vi "ROSNode.vi"(2 "Response":T1, 3 "ROS":T3={"topic port"=7000, "Node"="/LVROS", "topic"="/LVROS", "type"="", "node port"=7000, "error "={"status"=FALSE, "code"=0, "source"=""}, "Direction"=enum."Node", "Update (ms)"=1, "FIFO size"=1}) -> ()   [LabVIEW 2012]
doc: "Performs the functions of a ROS node: adds a publisher to the registered publisher list and registers with the master, starts and updates publishers, adds subscribers, and opens ports for subscribers and publishers"
uses:
  Console/Servers/ServerSubs/MyState.ctl
  _ROSDefinition.vi
  Console/Servers/ServerSubs/ROSLog.ctl
  <vilib>/Platform/browser.llb/Open URL in Default Browser (string).vi
  <vilib>/Utility/miscctls.llb/LVPointTypeDef.ctl
  SubVIs/_ROSDirection.ctl
  SubVIs/_ROSControl.ctl
panel:
  out "Color Code":picture
  out "Status out":T2[](array[typedef])
  out "Status":string
  out "Connections":bool
  out "Boundaries":cluster{i32, i32}[](array[cluster])=[{10, 22}, {30, 42}, {50, 62}]
  out "selection":i32=-1
  in  "HTML":bool
  out "ROS Master":string="130.64.16.138:11311"
  out "Registered":T3[](array[typedef])
  out "Last requestTopic":string
  out "Subscribers":T5(array[cluster])
  out "Queue log":string
  out "MyState":T2
  out "Setup":string
  in  "stop":bool
  out "HTML":picture
  out "Servers":picture
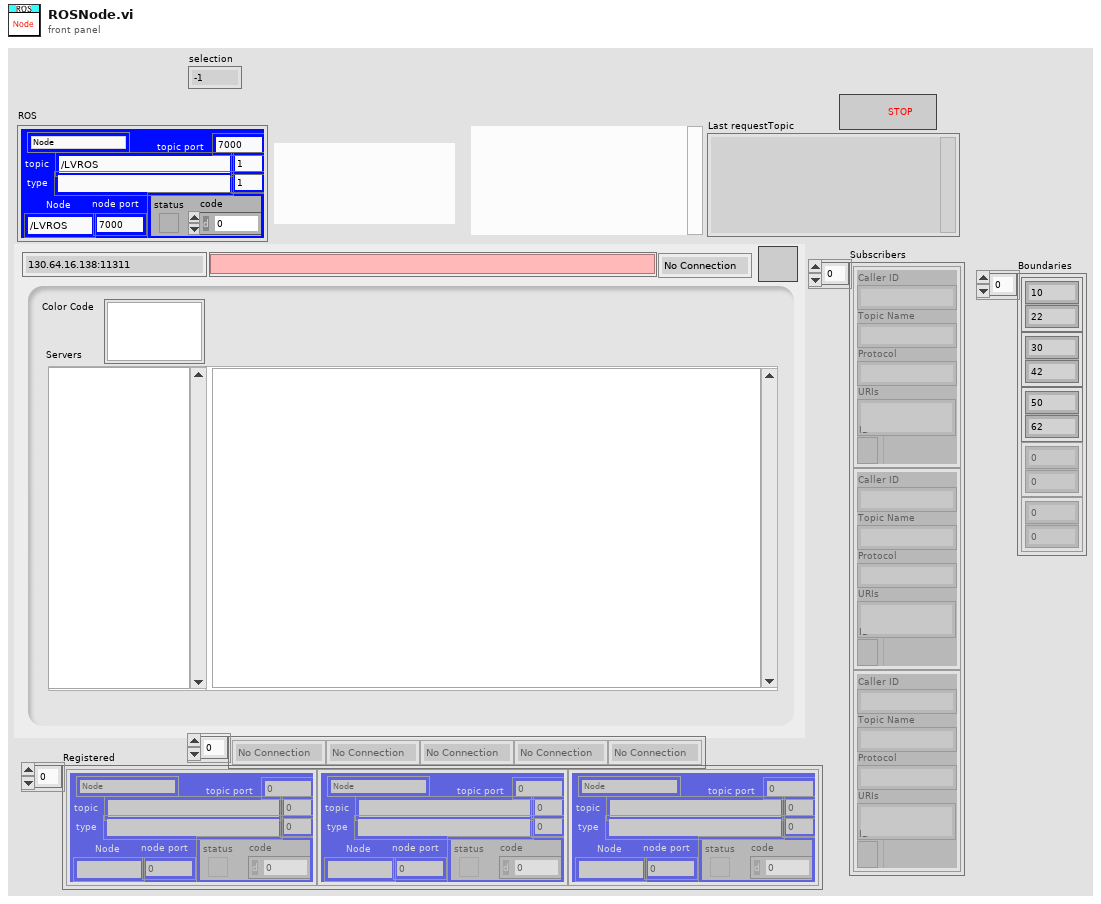
[diagram p1: front panel]
types:
  T1 = cluster{"Code":i32, "Status Message":string, "Nodes with this topic":string[]}
  T2 = typedef "MyState.ctl" = enum16{"No Connection", "Registered", "Connected", "Close"}
  T3 = typedef "_ROSControl.ctl" = cluster{"topic port":u16, "Node":string, "topic":string, "type":string, "node port":u16, "error ":errorcluster, "Direction":T4, "Update (ms)":u16, "FIFO size":u16}
  T4 = typedef "_ROSDirection.ctl" = enum16{"Node", "Publisher", "Subscriber", "ServiceClient", "ServiceProvider"}
  T5 = cluster{"Caller ID":string, "Topic Name":string, "Protocol":string, "URIs":string, "ID":refnum<k5>}[]
  T6 = enum16{"Reset Log", "Add Client", "Remove Client", "Add Task"}
  T7 = typedef "LVPointTypeDef.ctl" = cluster{"Horizontal":i16, "Vertical":i16}
  T8 = typedef "LVMouseTypeDef.ctl" = cluster{"Mouse Position":cluster{"X":i32, "Y":i32}, "Mouse Modifiers":cluster{"Button Down":bool, "Shift Mod":bool, "Menu Mod":bool, "Option Mod":bool}}
  T9 = cluster{"Caller ID":string, "Topic Name":string, "Node URIs":string[]}
  T10 = enum32{"Invalid", "Standard", "Closed", "Hidden", "Minimized", "Maximized"}
  T11 = typedef "ROSLog.ctl" = cluster{"Sent":string, "Reply":string, "MethodName":string, "success":bool, "Dir1":string, "Dir2":string, "Time Stamp":string, "error":errorcluster, "Preamble":string, "Midamble":string, "Postamble":string}
  T12 = cluster{"Caller ID":string, "Topic Name":string, "Protocol":string, "URI":string, "ID":refnum<k5>}
  T13 = cluster{"Caller ID":string, "Topic Name":string, "Protocol":string, "URI":string, "ID":refnum<k5>}[]
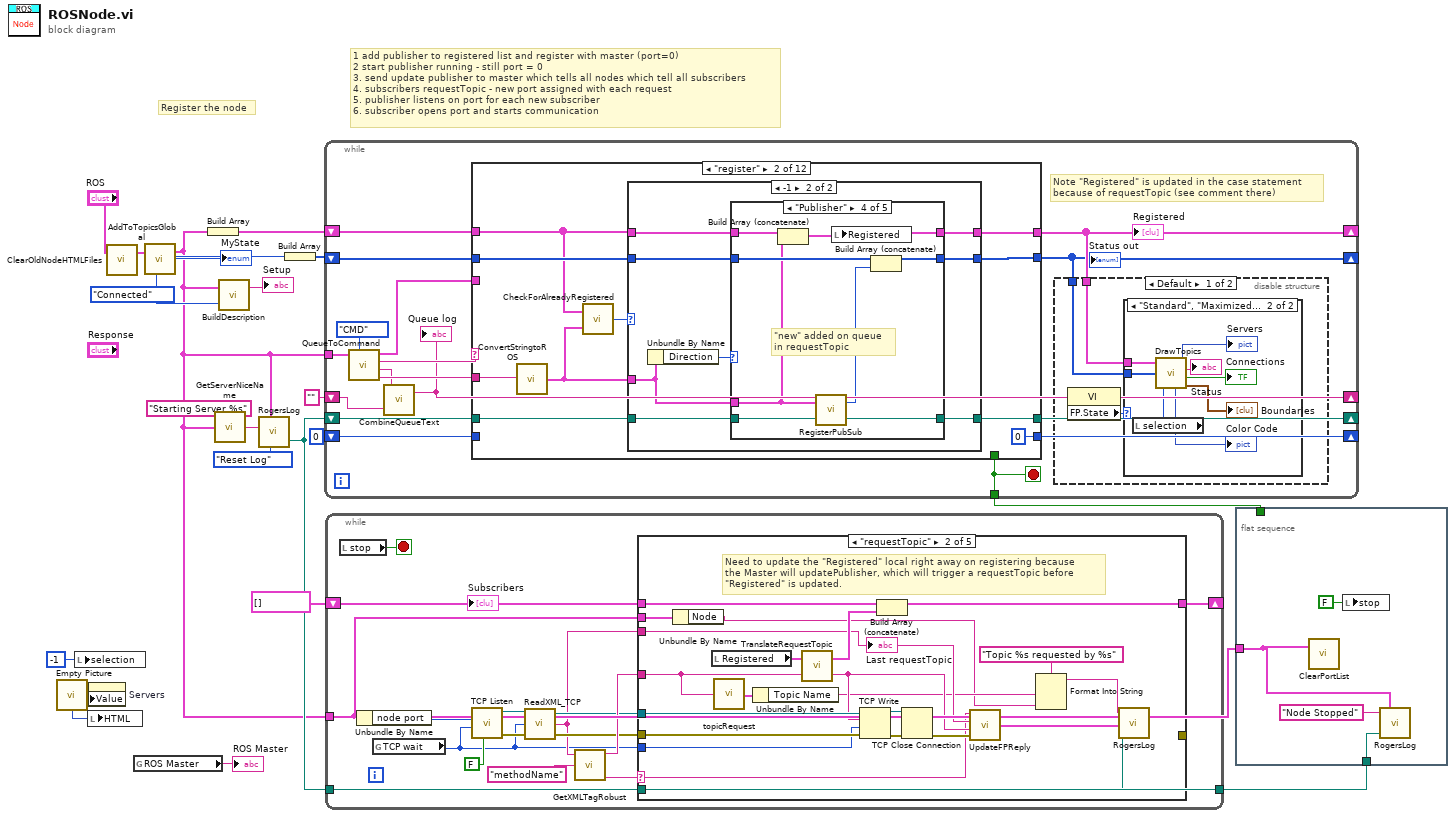
[diagram p0: block diagram]
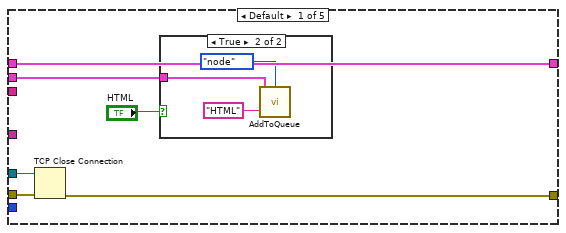
[diagram p2: hidden frame]
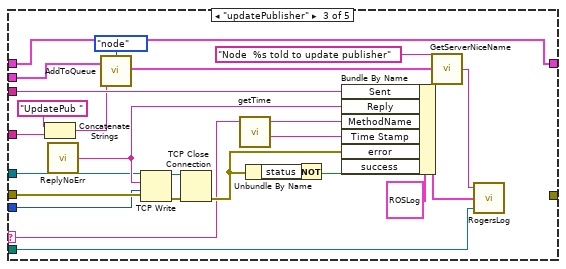
[diagram p4: hidden frame]
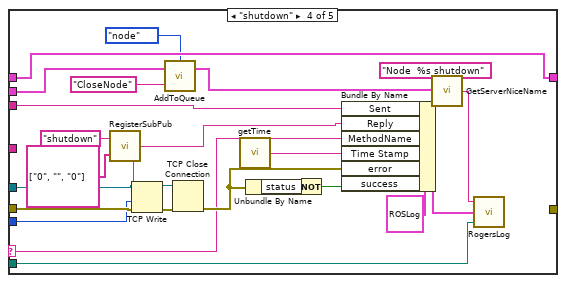
[diagram p5: hidden frame]
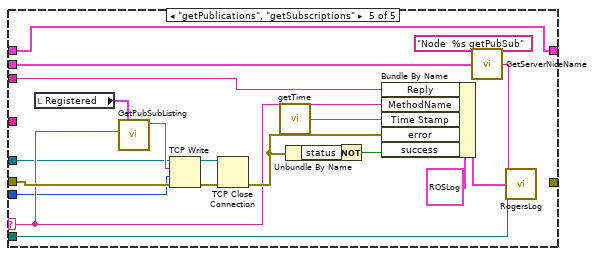
[diagram p6: hidden frame]
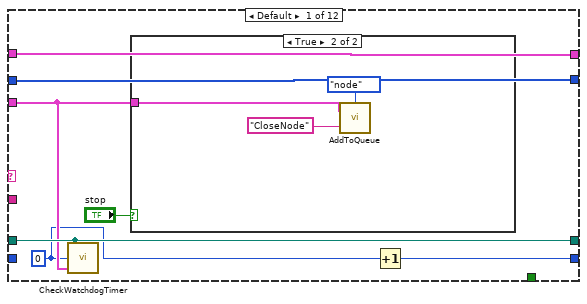
[diagram p9: hidden frame]
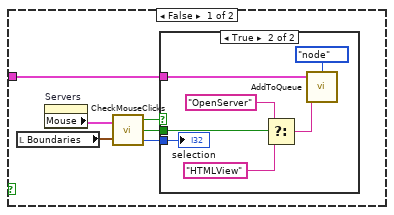
[diagram p10: hidden frame]
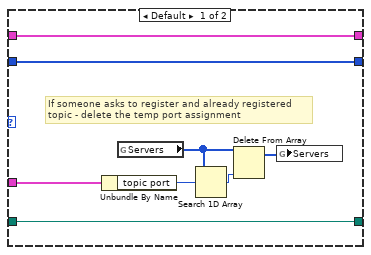
[diagram p12: hidden frame]
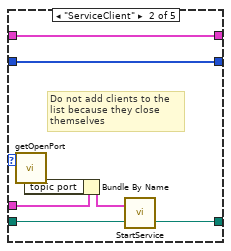
[diagram p14: hidden frame]
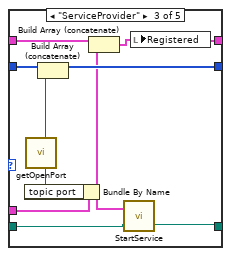
[diagram p15: hidden frame]
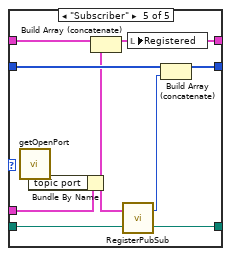
[diagram p16: hidden frame]
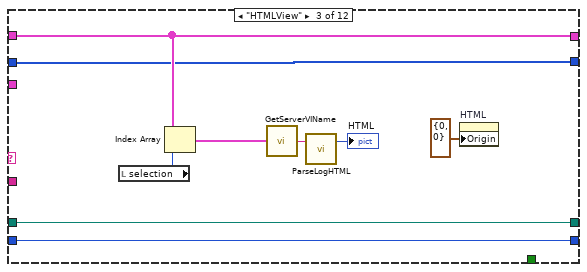
[diagram p17: hidden frame]
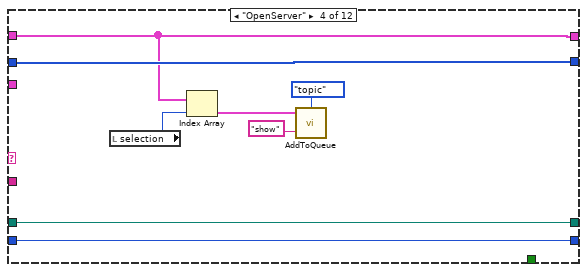
[diagram p18: hidden frame]
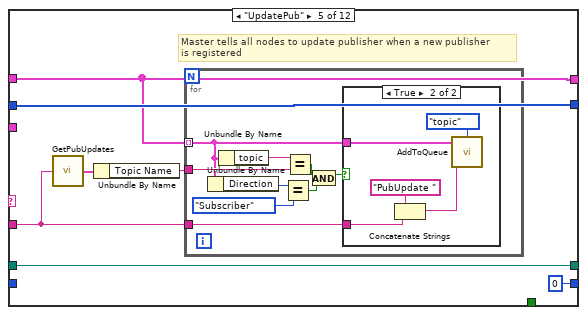
[diagram p19: hidden frame]
diagram:
  w12 = MyState."Connected" ("MyState")
  # "Register the node"
  # "1 add publisher to registered list and register with master (port=0)\n2 start publisher running - still port = 0\n3. send update publisher to master which tells all nodes which tell all subscribers\n4. subscribers requestTopic - new port assigned with each request\n5. publisher listens on port for each new subscriber\n6. subscriber opens port and starts communication"
  n1 = call "Empty Picture"() -> ("empty picture"=w10:picture)
  n2 = local write "selection"(-1 ("selection")) -> ()
  n3 = local write "HTML"(w10) -> ()
  n4 = property on="Servers" class="Pict"("Value"=w10) -> ()  [unwired: 2 in, 2 out]
  n5 = call "ClearOldNodeHTMLFiles.vi"("ROS"="ROS") -> ("ROS out"=w2:T3)  [unwired: 2 in]
  n6 = global read "_ROSDefinition.vi" "ROS Master"() -> (→"ROS Master":string)
  n7 = call "AddToTopicsGlobal.vi"("ROS in"=w2) -> ("ROS out"=w1:T3)  [unwired: 2 in]
  n8 = Build Array(w1) -> (w13:T3[])
  n9 = call "GetServerNiceName.vi"("ROS"=w1, "Text to add"="Starting Server %s") -> ("String"=w17:string)
  n10 = call "BuildDescription.vi"("MyState"=w12, "ROS in"=w1) -> ("Setup"=→"Setup":string)  [unwired: 1 in]
  n11 = call "RogersLog.vi"("Text to add"=w17, "ROS"=w1, "Task"=T6."Reset Log") -> ("LogPath out"=w7:path)  [unwired: 2 in, 1 out]
  n12 = Build Array(w12) -> (w11:T2[])
  n13 = while {
    tunnel: w1 -> [w30]
    tunnel: [w33] -> w14
    shift-right: [w29] -> _
    shift-left: w13 -> [w34]
    shift-right: [w31] -> _
    shift-left: w7 -> [w32]
    shift-right: [w27] -> _
    shift-left: w11 -> [w28]
    shift-right: [w25] -> _
    shift-left: 0 ("selection") -> [w26]
    shift-right: [w24] -> _
    shift-left: "" ("New List") -> [w23]
    stop <- w33 stop-if-true
    # "Note \"Registered\" is updated in the case statement\nbecause of requestTopic (see comment there)"
    n14 = call "QueueToCommand.vi"("ROS"=w30, "Check"=enum16{"Cmd+Write", "FIFO", "CMD", "CMD /wait"}."CMD") -> ("ROS out"=w21:T3, "Command"=w36:string, "Queue log"=w22:string, "data"=w35:string)  [unwired: 1 in]
    n15 = call "CombineQueueText.vi"("Old List"=w23, "Queue In"=w22) -> ("New List"=w24:string)  [unwired: 1 in]
    "Queue log" <- w24
    n16 = case shown="\"register\"" w36 {
      tunnel: w35 -> [_ w80 _ _ w152 w181 _ _ _ _ w239 _]
      tunnel: [w53 w79 w137 w148 w153 w175 w201 w209 w229 w233 w242 w261] -> w29
      tunnel: w34 -> [w53 w73 w137 w148 w153 w176 w202 w209 w229 w233 w242 w261]
      tunnel: [_ _ _ _ _ _ _ _ w226 _ _ _] -> w33
      tunnel: w32 -> [w51 w78 w139 w150 w157 w180 w204 w211 w227 w232 w248 w259]
      tunnel: [w51 w77 w139 w150 w157 w179 w204 w211 w227 w232 w248 w259] -> w31
      tunnel: w21 -> [w50 _ _ _ _ _ w196 w208 _ _ _ w257]
      tunnel: w28 -> [w52 w76 w135 w149 w156 w174 w200 w212 w228 w231 w245 w260]
      tunnel: [w52 w75 w135 w149 w156 w173 w199 w212 w228 w231 w244 w260] -> w27
      tunnel: w26 -> [_ _ w134 w146 _ _ _ _ w225 w230 _ w258]
      tunnel: [w49 0 w134 w146 0 0 0 0 w225 w230 0 ("selection") w258] -> w25
      frame Default {
        w48 = 0 ("selection")
        n17 = call "CheckWatchdogTimer.vi"("ROS"=w50, "itteration"=w48, "LogPath in"=w51) -> ()  [unwired: 3 in]
        n18 = case shown="True" "stop" {
          tunnel: w50 -> [w57 w69]
          frame False {
            n19 = local read "Boundaries"() -> (w56:cluster{i32, i32}[])
            n20 = property on="Servers" class="Pict"() -> ("Mouse"=w58:T8)  [unwired: 2 in, 2 out]
            n21 = call "CheckMouseClicks.vi"("Mouse"=w58, "Boundaries"=w56) -> ("Change?"=w59:bool, "Shift?"=w55:bool, "selection"=w60:i32)
            n22 = case shown="True" w59 {
              tunnel: w60 -> [_ w67]
              tunnel: w57 -> [_ w62]
              tunnel: w55 -> [_ w65]
              frame False {
              }
              frame True {
                n23 = Select(t="OpenServer" ("element"), s=w65, f="HTMLView" ("element")) -> (s? t:f=w63:string)
                n24 = call "AddToQueue.vi"("Cmd"=w63, "ROS"=w62, "Type"=enum16{"topic", "node", "ToFIFO", "ToWrite"}."node") -> ()  [unwired: 2 in, 1 out]
                "selection" <- w67
              }
            }
          }
          frame True {
            n25 = call "AddToQueue.vi"("Cmd"="CloseNode" ("element"), "ROS"=w69, "Type"=enum16{"topic", "node"}."node" ("Name")) -> ()  [unwired: 2 in, 1 out]
          }
        }
        n26 = Increment(x=w48) -> (x+1=w49:i32)
      }
      frame "register" {
        n27 = call "ConvertStringtoROS.vi"("string in"=w80) -> ("ROS"=w72:T3)
        n28 = call "CheckForAlreadyRegistered.vi"("ROS"=w72, "Registered"=w73) -> ("index of element"=w74:i32)
        n29 = case shown="-1" w74 {
          tunnel: w72 -> [w85 w89]
          tunnel: [w88 w96] -> w79
          tunnel: w73 -> [w88 w95]
          tunnel: w78 -> [w86 w94]
          tunnel: [w86 w93] -> w77
          tunnel: w76 -> [w87 w92]
          tunnel: [w87 w91] -> w75
          frame Default {
            # "If someone asks to register and already registered\ntopic - delete the temp port assignment"
            n30 = Unbundle By Name(w85) -> ("topic port"=w84:u16)
            n31 = global read "_ROSDefinition.vi" "Servers"() -> (w82:u16[])
            n32 = Search 1D Array(1D array=w82, element=w84) -> (index of element=w83:i32)  [unwired: 1 in]
            n33 = Delete From Array(array=w82, index=w83) -> (array with subset deleted=w81:u16[])  [unwired: 1 in, 1 out]
            n34 = global write "_ROSDefinition.vi" "Servers"(w81) -> ()
          }
          frame -1 {
            n35 = Unbundle By Name(w89) -> ("Direction"=w90:T4)
            n36 = case shown="\"Publisher\"" w90 {
              tunnel: [w99 w101 w112 w116 w124] -> w96
              tunnel: w95 -> [w99 w101 w114 w123 w133]
              tunnel: w94 -> [w97 w106 w108 w122 w132]
              tunnel: [w97 w105 w107 w121 w131] -> w93
              tunnel: w92 -> [w98 w100 w113 w120 w130]
              tunnel: [w98 w100 w111 w119 w129] -> w91
              tunnel: w89 -> [_ w103 w115 w117 w126]
              frame "Node", Default {
              }
              frame "ServiceClient" {
                # "Do not add clients to the \nlist because they close \nthemselves"
                n37 = call "getOpenPort.vi"() -> ("port"=w104:u16)
                n38 = Bundle By Name(cluster=w103, "topic port"=w104) -> (w102:T3)
                n39 = call "StartService.vi"("LogPath in"=w106, "New server ROS"=w102) -> ("LogPath out"=w105:path)  [unwired: 1 out]
              }
              frame "ServiceProvider" {
                n40 = call "getOpenPort.vi"() -> ("port"=w110:u16)
                n41 = Bundle By Name(cluster=w115, "topic port"=w110) -> (w109:T3)
                n42 = Build Array (concatenate)(w113, w110) -> (w111:u16[])
                n43 = Build Array (concatenate)(w114, w109) -> (w112:T3[])
                n44 = call "StartService.vi"("LogPath in"=w108, "New server ROS"=w109) -> ("LogPath out"=w107:path)  [unwired: 1 out]
                n45 = local write "Registered"(w112) -> ()
              }
              frame "Publisher" {
                # "\"new\" added on queue\nin requestTopic"
                n46 = Build Array (concatenate)(w123, w117) -> (w116:T3[])
                n47 = call "RegisterPubSub.vi"("LogPath in"=w122, "New server ROS"=w117) -> ("LogPath out"=w121:path, "MyState"=w118:T2)
                n48 = local write "Registered"(w116) -> ()
                n49 = Build Array (concatenate)(w120, w118) -> (w119:u16[])
              }
              frame "Subscriber" {
                n50 = call "getOpenPort.vi"() -> ("port"=w127:u16)
                n51 = Bundle By Name(cluster=w126, "topic port"=w127) -> (w125:T3)
                n52 = Build Array (concatenate)(w133, w125) -> (w124:T3[])
                n53 = call "RegisterPubSub.vi"("LogPath in"=w132, "New server ROS"=w125) -> ("LogPath out"=w131:path, "MyState"=w128:T2)
                n54 = local write "Registered"(w124) -> ()
                n55 = Build Array (concatenate)(w130, w128) -> (w129:u16[])
              }
            }
          }
        }
      }
      frame "HTMLView" {
        n56 = local read "selection"() -> (w140:i32)
        n57 = Index Array(array=w137, index=w140) -> (element=w136:T3)
        n58 = call "GetServerVIName.vi"("ROS"=w136) -> ("vi name"=w141:string)
        n59 = call "ParseLogHTML.vi"("vi name"=w141) -> ("2D Picture"=→"HTML":picture)  [unwired: 1 in, 1 out]
        n60 = property on="HTML" class="Pict"("Origin"=T7 {"Horizontal"=0, "Vertical"=0}) -> ()  [unwired: 2 in, 2 out]
      }
      frame "OpenServer" {
        n61 = local read "selection"() -> (w147:i32)
        n62 = Index Array(array=w148, index=w147) -> (element=w145:T3)
        n63 = call "AddToQueue.vi"("Cmd"="show" ("element"), "ROS"=w145, "Type"=enum16{"topic", "node", "ToFIFO", "ToWrite"}."topic") -> ()  [unwired: 2 in, 1 out]
      }
      frame "UpdatePub" {
        # "Master tells all nodes to update publisher when a new publisher\nis registered"
        n64 = call "GetPubUpdates.vi"("XML"=w152) -> ("PubUpdate"=w155:T9)
        n65 = Unbundle By Name(w155) -> ("Topic Name"=w154:string)
        n66 = for {
          tunnel: w153 -> [w159] mode=indexing
          tunnel: w154 -> [w165]
          tunnel: w152 -> [w158]
          n67 = Unbundle By Name(w159) -> ("Direction"=w164:T4)
          n68 = Unbundle By Name(w159) -> ("topic"=w166:string)
          n69 = Equal?(x=w164, y=_ROSDirection."Subscriber" ("Direction")) -> (x = y?=w161:bool)
          n70 = Equal?(x=w166, y=w165) -> (x = y?=w162:bool)
          n71 = And(x=w162, y=w161) -> (x .and. y?=w160:bool)
          n72 = case shown="True" w160 {
            tunnel: w159 -> [_ w168]
            tunnel: w158 -> [_ w170]
            frame False {
            }
            frame True {
              n73 = Concatenate Strings("PubUpdate " ("string"), w170) -> (w169:string)
              n74 = call "AddToQueue.vi"("Cmd"=w169, "ROS"=w168, "Type"=enum16{"topic", "node", "ToFIFO", "ToWrite"}."topic") -> ()  [unwired: 2 in, 1 out]
            }
          }
        }
      }
      frame "unregister" {
        n75 = call "ConvertStringtoROS.vi"("string in"=w181) -> ("ROS"=w178:T3)
        n76 = call "CheckForAlreadyRegistered.vi"("ROS"=w178, "Registered"=w176) -> ("index of element"=w177:i32)
        n77 = case shown="Default" w177 {
          selector: w177 -> [_ w188]
          tunnel: w180 -> [w182 w194]
          tunnel: [w182 w193] -> w179
          tunnel: w178 -> [_ w186]
          tunnel: w176 -> [w184 w187]
          tunnel: [w184 w191] -> w175
          tunnel: w174 -> [w183 w190]
          tunnel: [w183 w189] -> w173
          frame -1 {
          }
          frame Default {
            # "Stop Server"
            n78 = Delete From Array(array=w187, index=w188) -> (array with subset deleted=w191:T3[])  [unwired: 1 in, 1 out]
            n79 = Delete From Array(array=w190, index=w188) -> (array with subset deleted=w189:u16[])  [unwired: 1 in, 1 out]
            n80 = call "UnRegisterPubSub.vi"("LogPath in"=w194, "ROS"=w186) -> ("LogPath out"=w193:path)  [unwired: 1 out]
            n81 = call "AddToQueue.vi"("Cmd"="done" ("element"), "ROS"=w186, "Type"=enum16{"topic", "node"}."topic" ("Name")) -> ()  [unwired: 2 in, 1 out]
          }
        }
      }
      frame "shutdown" {
        # "Stop Server"
        n82 = call "CheckForAlreadyRegistered.vi"("ROS"=w196, "Registered"=w202) -> ("index of element"=w203:i32)
        n83 = call "AddToQueue.vi"("Cmd"="done" ("element"), "ROS"=w196, "Type"=enum16{"topic", "node"}."node" ("Name")) -> ()  [unwired: 2 in, 1 out]
        n84 = Delete From Array(array=w202, index=w203) -> (array with subset deleted=w201:T3[])  [unwired: 1 in, 1 out]
        n85 = Delete From Array(array=w200, index=w203) -> (array with subset deleted=w199:u16[])  [unwired: 1 in, 1 out]
      }
      frame "CloseNode" {
        n86 = for {
          tunnel: w209 -> [w216] mode=indexing
          tunnel: w208 -> [w214]
          tunnel: [w213] -> w206
          n87 = Unbundle By Name(w216) -> ("Direction"=w215:T4)
          n88 = case shown="Default" w215 {
            tunnel: w216 -> [_ w224]
            tunnel: w214 -> [w217 w221]
            tunnel: [w217 w218] -> w213
            frame "Node" {
              # "Provider closes in server\nand Node closes in \nshutdown."
            }
            frame Default {
              # "unregister Server"
              n89 = Flatten To String(anything=w224) -> (data string=w223:string)  [unwired: 3 in, 2 out]
              n90 = Concatenate Strings("unregister " ("element"), w223) -> (w220:string)
              n91 = call "AddToQueue.vi"("Cmd"=w220, "ROS"=w221, "Type"=enum16{"topic", "node"}."node" ("Name")) -> ("ROS out"=w218:T3)  [unwired: 2 in]
            }
          }
        }
        n92 = call "AddToQueue.vi"("Cmd"="shutdown" ("element"), "ROS"=w206, "Type"=enum16{"topic", "node"}."node" ("Name")) -> ()  [unwired: 2 in, 1 out]
      }
      frame "done" {
        w226 = TRUE ("stop")
        n93 = local write "stop"(w226) -> ()
      }
      frame "HTML" {
        n94 = disable-structure shown="Default" {
          disable-tunnel: w232 -> [w234 _]
          frame condition #0 (active) {
            n95 = call "GetLogFilePath.vi"() -> ("LogFolder"=w236:path)  [unwired: 2 in, 1 out]
            n96 = Build Path(base path=w236, name or relative path="index.html" ("pattern")) -> ()  [unwired: 1 out]
            n97 = call <vilib>:"Path to URL.vi"("path"=w234) -> ("url"=w237:string)
            n98 = call-poly <vilib>:"Open URL in Default Browser.vi"("URL"=w237) -> ()  [unwired: 5 in, 2 out]
          }
          frame condition #1 {
          }
        }
      }
      frame "status" {
        n99 = Match Pattern(string=w239, regular expression="STATE") -> (before substring=w243:string, after substring=w246:string)  [unwired: 1 in, 2 out]
        n100 = call "ConvertStringtoROS.vi"("string in"=w243) -> ("ROS"=w241:T3)
        n101 = call "CheckForAlreadyRegistered.vi"("ROS"=w241, "Registered"=w242) -> ("index of element"=w240:i32)
        n102 = case shown="Default" w240 {
          selector: w240 -> [w252 _]
          tunnel: w246 -> [w254 _]
          tunnel: w245 -> [w253 w255]
          tunnel: [w250 w255] -> w244
          frame Default {
            n103 = Scan From String(format string="%d", input string=w254) -> (output 1=w251:i32)  [unwired: 3 in, 3 out]
            n104 = Replace Array Subset(array=w253, new element=w251, index=w252) -> (w250:u16[])
          }
          frame -1 {
          }
        }
      }
      frame "show" {
        n105 = global read "_ROSDefinition.vi" "ROS Master"() -> (w256:string)
        n106 = local write "ROS"(w257) -> ()
        n107 = local write "ROS Master"(w256) -> ()
        n108 = control-ref of="This VI"() -> (w262:refnum<vi>)
        n109 = invoke class="VI" method="FP.Open"(reference=w262) -> ()  [unwired: 4 in, 5 out]
      }
    }
    "Registered" <- w29
    "Status out" <- w27
    n110 = disable-structure shown="Default" {
      disable-tunnel: w29 -> [w39 _]
      disable-tunnel: w27 -> [w38 _]
      frame condition #0 (active) {
        n111 = property class="VI"() -> ("FP.State"=w37:T10)  [unwired: 2 in, 2 out]
        n112 = case shown="\"Standard\", \"Maximized\"" w37 {
          tunnel: w39 -> [_ w42]
          tunnel: w38 -> [_ w41]
          frame "Invalid", Default {
          }
          frame "Standard", "Maximized" {
            n113 = local read "selection"() -> (w46:i32)
            n114 = call "DrawTopics.vi"("Registered"=w42, "Status"=w41, "Selection"=w46) -> ("new picture"=→"Servers":picture, "Status"=→"Status":string, "all good?"=→"Connections":bool, "Boundaries"=→"Boundaries":cluster{i32, i32}[], "Key"=→"Color Code":picture)
          }
        }
      }
      frame condition #1 {
      }
    }
  }
  n115 = while {
    shift-right: [w269] -> _
    shift-left: T5 [] ("Subscribers") -> [w270]
    tunnel: w1 -> [w264]
    tunnel: w7 -> [w263]
    tunnel: [w263] -> w4
    stop <- w278 stop-if-true
    n116 = local read "stop"() -> (w278:bool)
    n117 = Unbundle By Name(w264) -> ("node port"=w274:u16)
    n118 = global read "_ROSDefinition.vi" "TCP wait"() -> (w265:i32)
    n119 = call <vilib>:"TCP Listen.vi"("resolve remote address (T)"=FALSE, "timeout ms (wait forever: -1)"=w265, "port"=w274) -> ("error out"=w276:errorcluster, "connection ID"=w275:refnum<k5>)  [unwired: 4 in, 3 out]
    n120 = call "ReadXML_TCP.vi"("error in"=w276, "timeout ms (3000)"=w265, "connection ID in"=w275) -> ("error out"=w267:errorcluster, "data out"=w266:string, "connection ID out"=w268:refnum<k5>)
    n121 = call "GetXMLTagRobust.vi"("Tag"="methodName", "String"=w266) -> ("value"=w272:string, "String w/o Tag"=w271:string)  [unwired: 1 in, 2 out]
    n122 = case shown="\"requestTopic\"" w272 {
      selector: w272 -> [_ w297 w322 w352 w363]
      tunnel: w271 -> [_ w294 w319 _ _]
      tunnel: w270 -> [w284 w309 w320 w351 w370]
      tunnel: [w284 w308 w320 w351 w370] -> w269
      tunnel: w268 -> [w280 w305 w324 w341 w359]
      tunnel: w267 -> [w281 w304 w323 w343 w365]
      tunnel: w266 -> [_ w298 w325 w346 w371]
      tunnel: w265 -> [_ w301 w321 w338 w360]
      tunnel: w264 -> [w283 w289 w311 w337 w364]
      tunnel: w263 -> [_ w295 w314 w347 w366]
      tunnel: [w279 _ _ _ _] -> _
      frame Default {
        n123 = TCP Close Connection(connection ID=w280, error in (no error)=w281) -> (error out=w279:errorcluster)  [unwired: 1 in, 1 out]
        n124 = case shown="True" "HTML" {
          tunnel: w283 -> [_ w286]
          frame False {
          }
          frame True {
            n125 = call "AddToQueue.vi"("Cmd"="HTML" ("element"), "ROS"=w286, "Type"=enum16{"topic", "node", "ToFIFO", "ToWrite"}."node") -> ()  [unwired: 2 in, 1 out]
          }
        }
      }
      frame "requestTopic" {
        # "Need to update the \"Registered\" local right away on registering because\nthe Master will updatePublisher, which will trigger a requestTopic before\n\"Registered\" is updated."
        n126 = Unbundle By Name(w289) -> ("Node"=w288:string)
        n127 = local read "Registered"() -> (w303:T3[])
        n128 = call "topicRequest.vi"("XML"=w294) -> ("Subscriber"=w293:T12)
        n129 = Unbundle By Name(w293) -> ("Topic Name"=w292:string)
        n130 = call "TranslateRequestTopic.vi"("String w/o Tag"=w294, "Registered"=w303) -> ("XML"=w299:string, "New Sub"=w302:T12)
        n131 = TCP Write(connection ID=w305, data in=w299, error in (no error)=w304, 9:w301) -> (connection ID out=w307:refnum<k5>, error out=w306:errorcluster)  [unwired: 1 out]
        n132 = Build Array (concatenate)(w309, w302) -> (w308:T13)
        n133 = TCP Close Connection(connection ID=w307, error in (no error)=w306) -> (error out=w300:errorcluster)  [unwired: 1 in, 1 out]
        n134 = call "UpdateFPReply.vi"("error in (no error)"=w300, "Reply"=w299, "Sent"=w298, "method"=w297) -> ("Log"=w296:T11)
        n135 = Format Into String(format string="Topic %s requested by %s" ("Text to add"), w292, w288) -> (resulting string=w290:string)  [unwired: 2 in, 1 out]
        n136 = call "RogersLog.vi"("Text to add"=w290, "Log"=w296, "LogPath in"=w295) -> ()  [unwired: 2 in, 2 out]
        "Last requestTopic" <- w298
      }
      frame "updatePublisher" {
        n137 = Concatenate Strings("UpdatePub " ("string"), w319) -> (w312:string)
        n138 = call "ReplyNoErr.vi"() -> ("msg out"=w329:string)  [unwired: 1 in]
        n139 = call "AddToQueue.vi"("Cmd"=w312, "ROS"=w311, "Type"=enum16{"topic", "node", "ToFIFO", "ToWrite"}."node") -> ("ROS out"=w313:T3)  [unwired: 2 in]
        n140 = TCP Write(connection ID=w324, data in=w329, error in (no error)=w323, 9:w321) -> (connection ID out=w331:refnum<k5>, error out=w330:errorcluster)  [unwired: 1 out]
        n141 = TCP Close Connection(connection ID=w331, error in (no error)=w330) -> (error out=w328:errorcluster)  [unwired: 1 in, 1 out]
        n142 = call "getTime.vi"() -> ("Current Time"=w332:string)  [unwired: 1 in]
        n143 = Unbundle By Name(w328) -> ("status"=w327:bool)
        n144 = Not(x=w327) -> (.not. x?=w326:bool)
        n145 = Bundle By Name(cluster=T11 {"Sent"="", "Reply"="", "MethodName"="", "success"=TRUE, "Dir1"="From Master", "Dir2"="To Master", "Time Stamp"="", "error"={"status"=FALSE, "code"=0, "source"=""}, "Preamble"="", "Midamble"="", "Postamble"=""} ("Log"), "Sent"=w325, "Reply"=w329, "MethodName"=w322, "Time Stamp"=w332, "error"=w328, "success"=w326) -> (w317:T11)
        n146 = call "GetServerNiceName.vi"("ROS"=w313, "Text to add"="Node  %s told to update publisher") -> ("String"=w315:string)
        n147 = call "RogersLog.vi"("Text to add"=w315, "Log"=w317, "LogPath in"=w314) -> ()  [unwired: 2 in, 2 out]
      }
      frame "shutdown" {
        n148 = call "RegisterSubPub.vi"("Parameters"=string[] ["0", "", "0"], "MethodName"="shutdown") -> ("XML"=w340:string)
        n149 = TCP Write(connection ID=w341, data in=w340, error in (no error)=w343, 9:w338) -> (connection ID out=w339:refnum<k5>, error out=w342:errorcluster)  [unwired: 1 out]
        n150 = call "AddToQueue.vi"("Cmd"="CloseNode" ("element"), "ROS"=w337, "Type"=enum16{"topic", "node", "ToFIFO", "ToWrite"}."node") -> ("ROS out"=w335:T3)  [unwired: 2 in]
        n151 = TCP Close Connection(connection ID=w339, error in (no error)=w342) -> (error out=w355:errorcluster)  [unwired: 1 in, 1 out]
        n152 = call "getTime.vi"() -> ("Current Time"=w356:string)  [unwired: 1 in]
        n153 = Unbundle By Name(w355) -> ("status"=w354:bool)
        n154 = Not(x=w354) -> (.not. x?=w353:bool)
        n155 = Bundle By Name(cluster=T11 {"Sent"="", "Reply"="", "MethodName"="", "success"=TRUE, "Dir1"="From Master", "Dir2"="To Master", "Time Stamp"="", "error"={"status"=FALSE, "code"=0, "source"=""}, "Preamble"="", "Midamble"="", "Postamble"=""} ("Log"), "Sent"=w346, "Reply"=w340, "MethodName"=w352, "Time Stamp"=w356, "error"=w355, "success"=w353) -> (w350:T11)
        n156 = call "GetServerNiceName.vi"("ROS"=w335, "Text to add"="Node  %s shutdown") -> ("String"=w348:string)
        n157 = call "RogersLog.vi"("Text to add"=w348, "Log"=w350, "LogPath in"=w347) -> ()  [unwired: 2 in, 2 out]
      }
      frame "getPublications", "getSubscriptions" {
        n158 = local read "Registered"() -> (w361:T3[])
        n159 = call "GetPubSubListing.vi"("Method"=w363, "Registered"=w361) -> ("StatusMessage"=w362:string)  [unwired: 9 in]
        n160 = TCP Write(connection ID=w359, data in=w362, 9:w360) -> (connection ID out=w358:refnum<k5>)  [unwired: 1 in, 2 out]
        n161 = TCP Close Connection(connection ID=w358, error in (no error)=w365) -> (error out=w374:errorcluster)  [unwired: 1 in, 1 out]
        n162 = call "getTime.vi"() -> ("Current Time"=w375:string)  [unwired: 1 in]
        n163 = Unbundle By Name(w374) -> ("status"=w373:bool)
        n164 = Not(x=w373) -> (.not. x?=w372:bool)
        n165 = Bundle By Name(cluster=T11 {"Sent"="", "Reply"="", "MethodName"="", "success"=TRUE, "Dir1"="From Master", "Dir2"="To Master", "Time Stamp"="", "error"={"status"=FALSE, "code"=0, "source"=""}, "Preamble"="", "Midamble"="", "Postamble"=""} ("Log"), "Reply"=w371, "MethodName"=w363, "Time Stamp"=w375, "error"=w374, "success"=w372) -> (w369:T11)
        n166 = call "GetServerNiceName.vi"("ROS"=w364, "Text to add"="Node  %s getPubSub") -> ("String"=w367:string)
        n167 = call "RogersLog.vi"("Text to add"=w367, "Log"=w369, "LogPath in"=w366) -> ()  [unwired: 2 in, 2 out]
      }
    }
    "Subscribers" <- w270
  }
  n168 = flat-sequence {
    tunnel: w14 -> [_]
    tunnel: w4 -> [w378]
    tunnel: w1 -> [w377]
    frame #0 {
      n169 = call "ClearPortList.vi"("ROS"=w377) -> ()  [unwired: 2 in]
      n170 = local write "stop"(FALSE ("stop")) -> ()
      n171 = call "RogersLog.vi"("Text to add"="Node Stopped", "ROS"=w377, "LogPath in"=w378) -> ()  [unwired: 2 in, 2 out]
    }
  }
  "MyState" <- w12
